vi "LEAPread.vi"(8 "error in (no error)":errorcluster, 11 "Controller Refnum In":refnum<k24>) -> (0 "error out":errorcluster, 1 "IsConnected":bool, 2 "Frame":T1, 3 "Controller Refnum Out":refnum<k24>)   [LabVIEW 2017, in "LeapMotion.lvlib"]
uses:
  LeapMotion.lvlib
  C:/Users/snordinh/Desktop/LEAP-sign-language-test/LEAP-sign-language-test/LeapMotion/Dynamic Libraries/LeapCSharp.NET4.5.dll
  Dynamic Libraries/LeapCSharp.NET4.5.dll
  TypeDefs/LEAPframe.ctl
  TypeDefs/LEAPhand.ctl
  TypeDefs/LEAPvector.ctl
  TypeDefs/LEAPfinger.ctl
  TypeDefs/LEAPbone.ctl
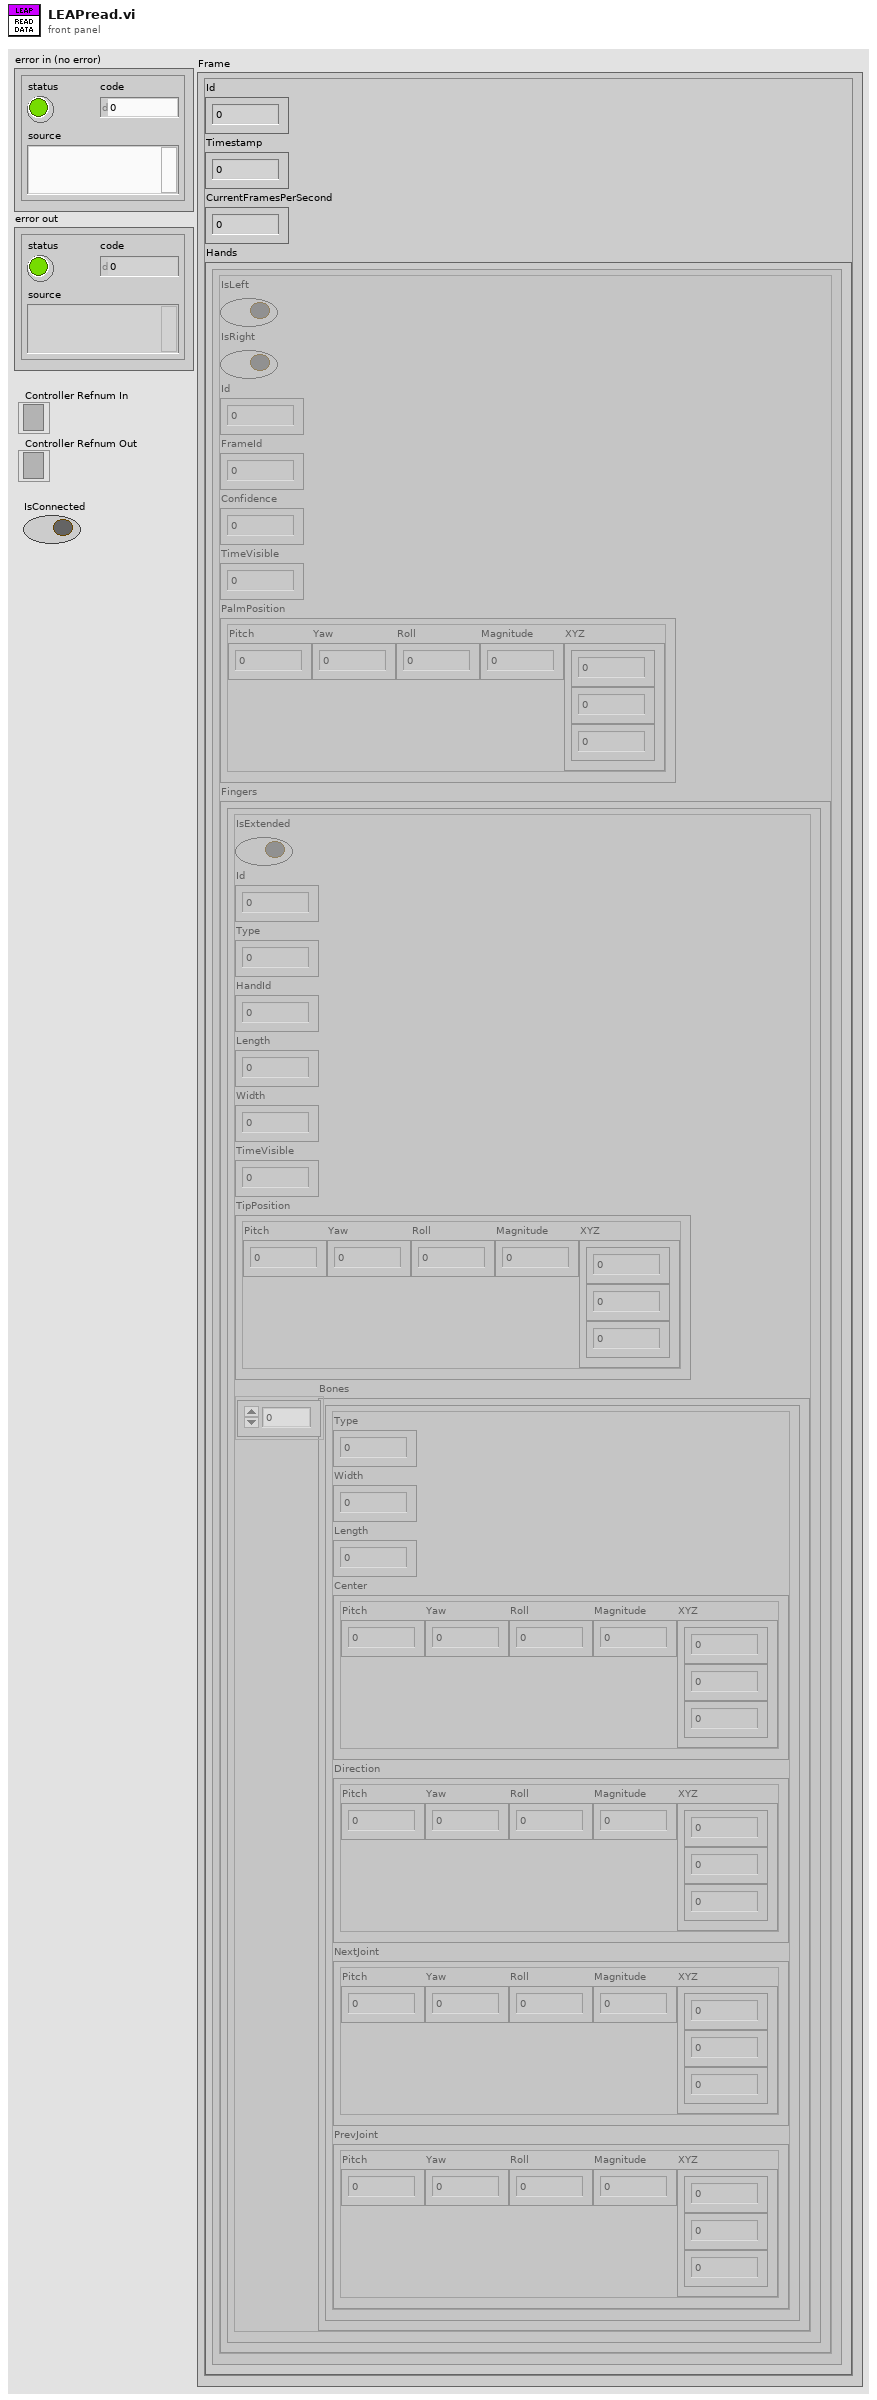
[diagram p1: front panel]
types:
  T1 = typedef "LeapMotion.lvlib/LEAPframe.ctl" = cluster{"Id":i64, "Timestamp":i64, "CurrentFramesPerSecond":sgl, "Hands":T2[]}
  T2 = typedef "LeapMotion.lvlib/LEAPhand.ctl" = cluster{"IsLeft":bool, "IsRight":bool, "Id":i32, "FrameId":i64, "Confidence":sgl, "TimeVisible":sgl, "PalmPosition":T3, "Fingers":T4[]}
  T3 = typedef "LeapMotion.lvlib/LEAPvector.ctl" = cluster{"Pitch":sgl, "Yaw":sgl, "Roll":sgl, "Magnitude":sgl, "XYZ":sgl[]}
  T4 = typedef "LeapMotion.lvlib/LEAPfinger.ctl" = cluster{"IsExtended":bool, "Id":i32, "Type":i32, "HandId":i32, "Length":sgl, "Width":sgl, "TimeVisible":sgl, "TipPosition":T3, "Bones":T5[]}
  T5 = typedef "LeapMotion.lvlib/LEAPbone.ctl" = cluster{"Type":i32, "Width":sgl, "Length":sgl, "Center":T3, "Direction":T3, "NextJoint":T3, "PrevJoint":T3}
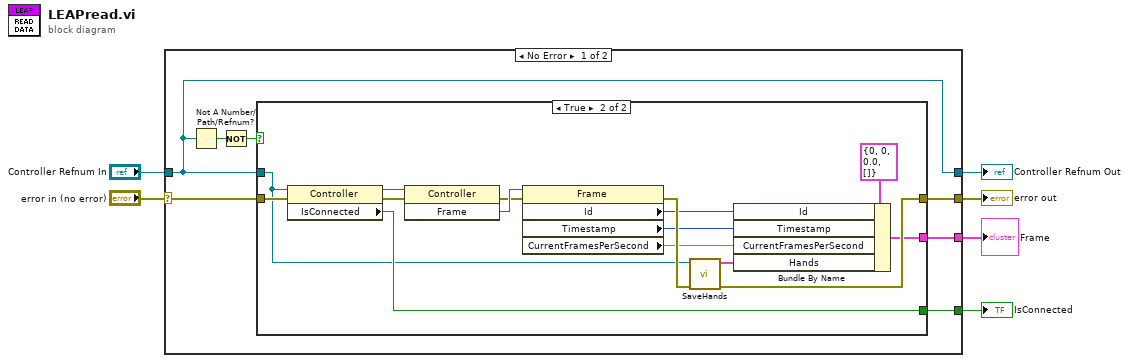
[diagram p0: block diagram]
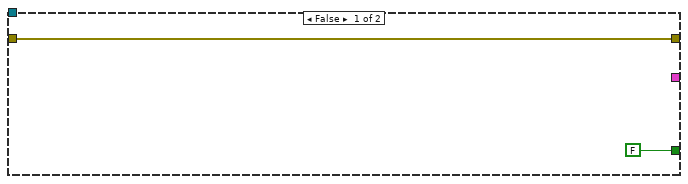
[diagram p2: hidden frame]
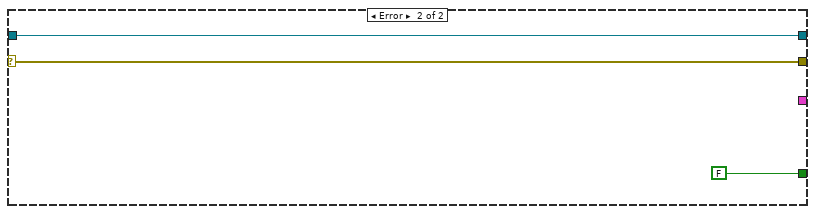
[diagram p3: hidden frame]
diagram:
  n1 = case shown="No Error" "error in (no error)" {
    selector: "error in (no error)" -> [w11 w32]
    tunnel: "Controller Refnum In" -> [w7 w31]
    tunnel: [w7 w31] -> w4
    tunnel: [w10 FALSE ("IsConnected")] -> w5
    tunnel: [w9 w32] -> w6
    tunnel: [w8 _] -> w1
    frame No Error {
      n2 = Not A Number/Path/Refnum?(number/path/refnum=w7) -> (NaN/Path/Refnum?=w13:bool)
      n3 = Not(x=w13) -> (.not. x?=w12:bool)
      n4 = case shown="True" w12 {
        tunnel: w11 -> [w14 w30]
        tunnel: w7 -> [_ w16]
        tunnel: [FALSE ("IsConnected") w27] -> w10
        tunnel: [w14 w23] -> w9
        tunnel: [_ w17] -> w8
        frame False {
        }
        frame True {
          n5 = property class="Controller"(reference=w16, error in=w30) -> (reference out=w28:refnum<k24>, error out=w29:errorcluster, "IsConnected"=w27:bool)
          n6 = invoke class="Controller" method="Frame"(reference=w28, error in=w29) -> (error out=w25:errorcluster, "Frame"=w26:refnum<k24>)  [unwired: 1 in, 1 out]
          n7 = property class="Frame"(reference=w26, error in=w25) -> (error out=w24:errorcluster, "Id"=w20:i64, "Timestamp"=w19:i64, "CurrentFramesPerSecond"=w18:sgl)  [unwired: 1 out]
          n8 = call "SaveHands.vi"("error in (no error)"=w24, "Leap.Controller"=w16) -> ("error out"=w23:errorcluster, "Hand array"=w21:T2[])  [unwired: 8 in]
          n9 = Bundle By Name(cluster=T1 {"Id"=0, "Timestamp"=0, "CurrentFramesPerSecond"=0.0, "Hands"=[]} ("Frame"), "Id"=w20, "Timestamp"=w19, "CurrentFramesPerSecond"=w18, "Hands"=w21) -> (w17:T1)
        }
      }
    }
    frame Error {
    }
  }
  "error out" <- w6
  "IsConnected" <- w5
  "Controller Refnum Out" <- w4
  "Frame" <- w1
